vi "cambiarcolor.vi"() -> ()   [LabVIEW 2016]
panel:
  in  "Stop Button":bool
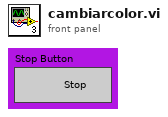
[diagram p1: front panel]
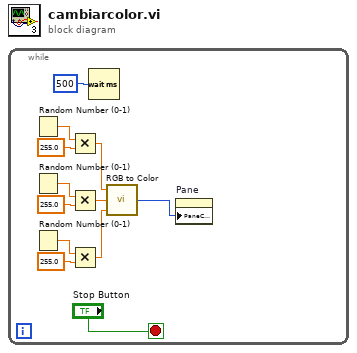
[diagram p0: block diagram]
diagram:
  n1 = while {
    stop <- "Stop Button" stop-if-true
    n2 = Random Number (0-1)() -> (number: 0 to 1=w4:dbl)
    n3 = Random Number (0-1)() -> (number: 0 to 1=w7:dbl)
    n4 = Random Number (0-1)() -> (number: 0 to 1=w8:dbl)
    n5 = Multiply(x=w4, y=255.0) -> (x*y=w10:dbl)
    n6 = Multiply(x=w7, y=255.0) -> (x*y=w11:dbl)
    n7 = Multiply(x=w8, y=255.0) -> (x*y=w12:dbl)
    n8 = Wait (ms)(milliseconds to wait=u32 500) -> ()  [unwired: 1 out]
    n9 = call <vilib>:"RGB to Color.vi"("B"=w12, "G"=w11, "R"=w10) -> ("Color"=w1:u32)
    n10 = property on="Pane" class="Pane"("PaneColor"=w1) -> ()  [unwired: 2 in, 2 out]
  }
